vi "switchToStreamMode.vi"(8 "error in (no error)":errorcluster, 10 "Stream Mode Algorithm":T1, 11 "Context in":refnum<class "Context.lvclass">) -> (0 "error out":errorcluster, 3 "Context out":refnum<class "Context.lvclass">)   [LabVIEW 2013, in "Context.lvclass"]
uses:
  Context.lvclass
  Configuration/Stream Mode Algorithm.ctl
  Context.lvclass/Context.ctl
  State/State.lvclass
  Model/Model/Model.lvclass
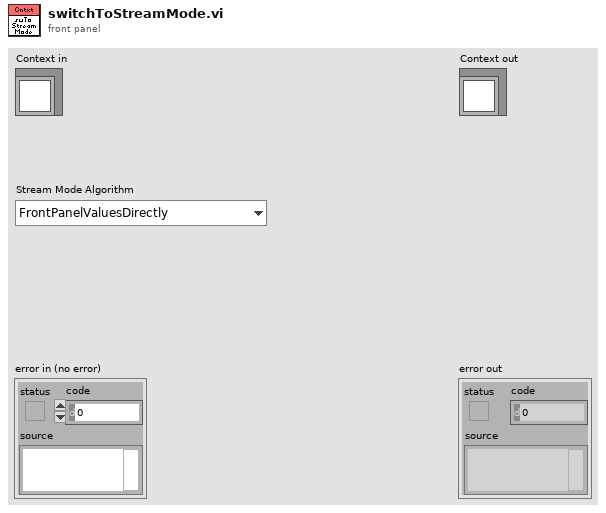
[diagram p1: front panel]
types:
  T1 = typedef "Stream Mode Algorithm.ctl" = enum16{"FrontPanelValuesDirectly"}
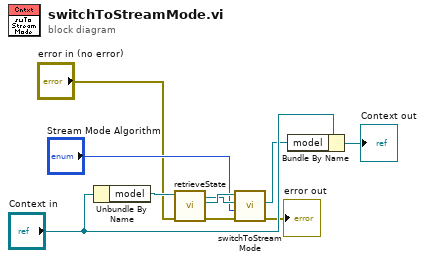
[diagram p0: block diagram]
diagram:
  n1 = Unbundle By Name("Context in") -> ("model"=w9:refnum<class "Model.lvclass">)
  n2 = call "retrieveState.vi"("error in (no error)"="error in (no error)", "Model in"=w9) -> ("error out"=w1:errorcluster, "state"=w10:refnum<class "State.lvclass">, "Model out"=w8:refnum<class "Model.lvclass">)  [unwired: 7 in]
  n3 = call-dynamic "switchToStreamMode.vi"("error in (no error)"=w1, "Stream Mode Algorithm"="Stream Mode Algorithm", "model"=w8, "State in"=w10) -> ("error out"=→"error out":errorcluster, "model 2"=w5:refnum<class "Model.lvclass">)  [unwired: 5 in, 1 out]
  n4 = Bundle By Name(cluster="Context in", "model"=w5) -> (→"Context out":refnum<class "Context.lvclass">)
